vi "Convert Message.vi"(8 "error in (no error)":errorcluster, 11 "Supporting PIDs in":refnum<class "Supported PIDs.lvclass">) -> (0 "error out":errorcluster, 1 "variant":variant, 2 "Result":dbl, 3 "Supporting PIDs out":refnum<class "Supported PIDs.lvclass">)   [LabVIEW 2011, in "Supported PIDs.lvclass"]
uses:
  Supported PIDs.lvclass
  Supported PIDs.lvclass/Supported PIDs.ctl
  PID.lvclass
panel:
  in  "Response In":string
  out "spreadsheet string":string
  out "Array":i32[](array[numeric])
  out "Boolean array":bool[](array[boolean])
  out "number":u32
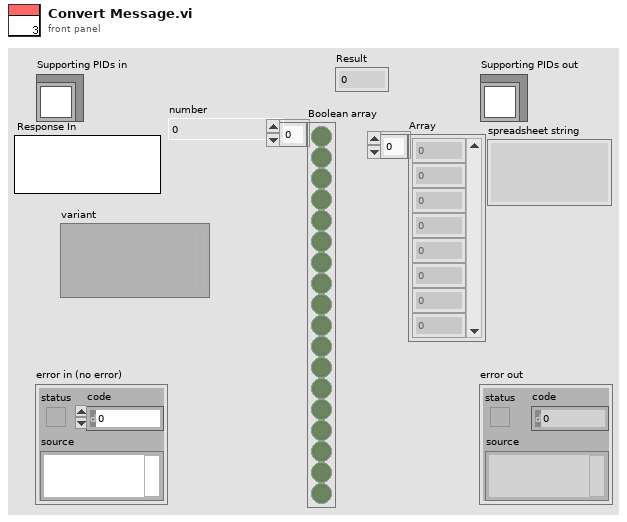
[diagram p1: front panel]
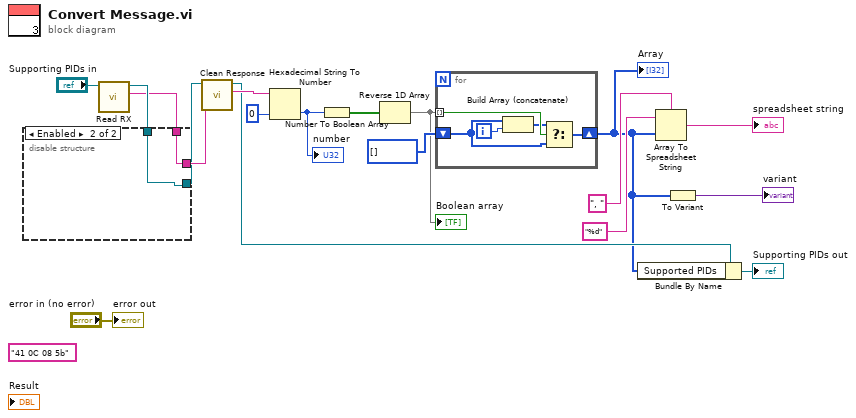
[diagram p0: block diagram]
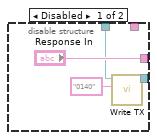
[diagram p2: hidden frame]
diagram:
  (unwired) "41 0C 08 5b" ("regular expression")
  n1 = call "Read RX.vi"("PID in"="Supporting PIDs in") -> ("RX"=w2:string, "PID out"=w4:refnum<class "Supported PIDs.lvclass">)  [unwired: 8 in, 1 out]
  n2 = disable-structure shown="Enabled" {
    disable-tunnel: ["Response In" w24] -> w5
    disable-tunnel: w4 -> [w22 w25]
    disable-tunnel: [w21 w25] -> w3
    disable-tunnel: w2 -> [_ w24]
    frame Disabled {
      n3 = call "Write TX.vi"("TX"="0140", "PID in"=w22) -> ("PID out"=w21:refnum<class "Supported PIDs.lvclass">)  [unwired: 8 in, 1 out]
    }
    frame Enabled {
    }
  }
  n4 = call-dynamic "Clean Response.vi"("Response In"=w5, "PID.lvclass"=w3) -> ("result string"=w17:string, "PID.lvclass 2"=w8:refnum<class "Supported PIDs.lvclass">)  [unwired: 7 in, 1 out]
  n5 = Hexadecimal String To Number(string=w17, default (0uL)=u32 0 ("default (0 U32)")) -> (number=w14:u32)  [unwired: 1 in, 1 out]
  "number" <- w14
  n6 = Number To Boolean Array(number=w14) -> (Boolean array=w15:bool[])
  n7 = Reverse 1D Array(array=w15) -> (reversed array=w13:bool[])
  "Boolean array" <- w13
  n8 = for {
    tunnel: w13 -> [w30] mode=indexing
    shift-right: [w26] -> w6
    shift-left: i32[] [] -> [w28]
    i -> [w29]
    n9 = Build Array (concatenate)(w28, w29) -> (w27:i32[])
    n10 = Select(t=w27, s=w30, f=w28) -> (s? t:f=w26:i32[])
  }
  "Array" <- w6
  n11 = Bundle By Name(cluster=w8, "Supported PIDs"=w6) -> (→"Supporting PIDs out":refnum<class "Supported PIDs.lvclass">)
  n12 = Array To Spreadsheet String(delimiter (Tab)=", ", array=w6, 3:"%d" ("format string")) -> (spreadsheet string=→"spreadsheet string":string)
  n13 = To Variant(anything=w6) -> (Variant=→"variant":variant)
  "error out" <- "error in (no error)"
